vi "Periodic Tasks.vi"(8 "error in":errorcluster) -> ()   [LabVIEW 2015]
doc: "This VI runs in parallel to other tasks. It can contain as many user-defined periodic loops as you need. These can carry out PID or other sorts of timed response."
uses:
  Device Refnums.ctl
  Drive Base - Controlled Mode - TypeDef.ctl
  Drive Base Mode.ctl
  Shooter Control.ctl
  Arm Mode TypeDef.ctl
  <vilib>/Rock Robotics/WPI/Solenoid/WPI_SolenoidValue.ctl
  Operator-Interface-Control-Board.git/trunk/LabVIEW/LED_Output_TypeDef.ctl
  Operator-Interface-Control-Board.git/trunk/LabVIEW/PWM_Output_TypeDef.ctl
  <vilib>/Rock Robotics/WPI/CAN/TalonSRX/WPI_CANTalonSRX_APIControlMode.ctl
  <vilib>/Rock Robotics/WPI/Utilities/WPI_GetSetVariantRefNum.vi
  Global Variables.vi
  <vilib>/Rock Robotics/Network Tables/NT Write Number.vi
  <vilib>/Rock Robotics/Network Tables/NT Read Number.vi
  <vilib>/addons/control/pid/pid.llb/PID (DBL).vi
  <vilib>/Rock Robotics/Network Tables/NT Write Numeric Array.vi
  <vilib>/Rock Robotics/WPI/Solenoid/WPI_SolenoidSetEnum.vi
  <vilib>/Rock Robotics/Network Tables/NT Write String.vi
  <vilib>/Rock Robotics/Network Tables/NT Write Boolean.vi
  <vilib>/Rock Robotics/WPI/Ultrasonic/WPI_SonarMB1010DigitalRefNum Registry Get.vi
  <vilib>/Rock Robotics/WPI/Ultrasonic/WPI_SonarMB1010DigitalGetRange.vi
  <vilib>/Utility/config.llb/Read Key (String).vi
  <vilib>/Utility/config.llb/Read Key (Boolean).vi
  <vilib>/Utility/config.llb/Read Key (Double).vi
  <vilib>/Rock Robotics/Network Tables/NT Write Raw.vi
  <vilib>/Rock Robotics/Network Tables/NT Write Boolean Array.vi
  <vilib>/Rock Robotics/Network Tables/NT Write String Array.vi
  ADIS16448-RoboRIO-Driver.git/trunk/LabVIEW/ADI MXP IMU/FRC ADI MXP IMU.lvlib
  <vilib>/addons/control/pid/NI_PID_pid.lvlib
  <vilib>/Utility/config.llb/NI_LVConfig.lvlib
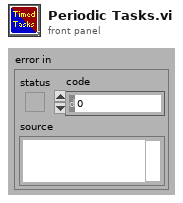
[diagram p1: front panel]
types:
  T1 = typedef "Device Refnums.ctl" = string
  T2 = typedef "Shooter Control.ctl" = cluster{"Fire":bool, "Open Claw":bool}
  T3 = typedef "Drive Base Mode.ctl" = enum16{"Disabled", "Controlled - Arcade", "Controlled - Tank", "Braked", "GRIP", "Encoder", "IMU", "Distance"}
  T4 = typedef "Drive Base - Controlled Mode - TypeDef.ctl" = cluster{"Drive Base Mode":T3, "Arcade":cluster{"y":dbl, "x":dbl}, "Tank":cluster{"Left":dbl, "Right":dbl}, "Target Encoder Value":cluster{"Left":dbl, "Right":dbl}, "Target IMU Angle":dbl, "Distance":dbl, "Target GRIP Area":dbl}
  T5 = typedef "WPI_EncoderDevRef.ctl" = cluster{"DevStatus":errorcluster, "EncoderIndex":T6, "CounterIndex":T7, "DistancePerCount":dbl, "Decoding Type":T8}
  T6 = typedef "FPGA_EncoderIdx.ctl" = enum8{"Enc 0", "Enc 1", "Enc 2", "Enc 3", "Enc 4", "Enc 5", "Enc 6", "Enc 7", "Invalid"}
  T7 = typedef "FPGA_CounterCtrSystemIndex.ctl" = enum8{"Ctr 0", "Ctr 1", "Ctr 2", "Ctr 3", "Ctr 4", "Ctr 5", "Ctr 6", "Ctr 7", "Invalid"}
  T8 = typedef "WPI_EncoderType.ctl" = enum16{"1x", "2x", "4x"}
  T9 = typedef "WPI_RobotDriveDevRef.ctl" = cluster{"DevStatus":errorcluster, "Motors[]":T10[], "Square Inputs":bool, "Max Output":dbl}
  T10 = typedef "WPI_MotorControlDeviceRef.ctl" = cluster{"DeviceStatus":errorcluster, "Type":T11, "PWM":cluster{"PWM Channel":T12, "DeadBand":T13}, "CAN":cluster{"Device Number":u8, "Control Mode":T14, "Semaphore":T15, "Max Vout":dbl, "TalonSRX Control Mode":T16}, "Invert":bool}
  T11 = typedef "WPI_MotorControlType.ctl" = enum16{"PWM", "CAN", "CANTalonSRX"}
  T12 = typedef "FPGA_DIOPWMChannel.ctl" = enum8{"PWM 0", "PWM 1", "PWM 2", "PWM 3", "PWM 4", "PWM 5", "PWM 6", "PWM 7", "PWM 8", "PWM 9", "PWM MXP 0", "PWM MXP 1", "PWM MXP 2", "PWM MXP 3", "PWM MXP 4", "PWM MXP 5", "PWM MXP 6", "PWM MXP 7", "PWM MXP 8", "PWM MXP 9", "Invalid"}
  T13 = typedef "WPI_PWMDeadband.ctl" = cluster{"Name":string, "maxPositivePwm":i32, "minPositivePwm":i32, "centerPwm":i32, "maxNegativePwm":i32, "minNegativePwm":i32, "angularRange":u16}
  T14 = typedef "WPI_CANJaguar_ControlMode.ctl" = enum8{"Percent VBus", "Current", "Speed", "Position", "Voltage"}
  T15 = typedef "Semaphore RefNum" = refnum<k1>
  T16 = typedef "WPI_CANTalonSRX_APIControlMode.ctl" = enum8{"Percent VBus", "Speed", "Position", "Slave", "Unchanged / Invalid", "Voltage Compensation", "Current", "Motion Profile"}
  T17 = typedef "WPI_SonarMB1010DigitalDeviceRef.ctl" = cluster{"CounterDevRef":T18, "Scaling factor (s/in)":dbl}
  T18 = typedef "WPI_CounterDevRef.ctl" = cluster{"DevStatus":errorcluster, "CntIndex":T7}
  T19 = typedef "FRC ADI MXP IMU.lvlib/WPI_AnalogDevicesIMUInterruptDevRef.ctl" = cluster{"SimpleGyroDevRef":T20, "InterruptRef":T22}
  T20 = typedef "FRC ADI MXP IMU.lvlib/WPI_AnalogDevicesIMUDevRef.ctl" = cluster{"DevStatus":errorcluster, "Handle":i32, "SPI Bus":T21, "Device Found":bool, "Sample Rate":dbl, "Device Ready":bool, "Yaw Axis":enum16{"X", "Y", "Z"}, "AHRS Algorithm":enum16{"Complementary", "Madgwick"}}
  T21 = typedef "spi_bus.ctl" = enum16{"SPI On-Board, CS0", "SPI On-Board, CS1", "SPI On-Board, CS2", "SPI On-Board, CS3", "SPI MXP", "Invalid"}
  T22 = typedef "WPI_InterruptRef.ctl" = cluster{"DevStatus":errorcluster, "InterruptIndex":T23}
  T23 = typedef "FPGA_InterruptIndex.ctl" = enum8{"0", "1", "2", "3", "4", "5", "6", "7", "Invalid"}
  T24 = typedef "WPI_AnalogChannelDevRef.ctl" = cluster{"DevStatus":errorcluster, "Analog Channel":T25}
  T25 = typedef "FPGA_AIChannel.ctl" = enum8{"AI 0", "AI 1", "AI 2", "AI 3", "AI MXP 0", "AI MXP 1", "AI MXP 2", "AI MXP 3", "Invalid"}
  T26 = typedef "Switch_Input_TypeDef.ctl" = cluster{"SW 0":bool, "SW 1":bool, "SW 2":bool, "SW 3":bool, "SW 4":bool, "SW 5":bool, "SW 6":bool, "SW 7":bool, "SW 8":bool, "SW 9":bool, "SW 10":bool, "SW 11":bool, "SW 12":bool, "SW 13":bool, "SW 14":bool, "SW 15":bool}
  T27 = typedef "GRIP Contours Report.ctl" = cluster{"area":dbl, "centerX":dbl, "centerY":dbl, "width":dbl, "height":dbl, "solidity":dbl}
  T28 = cluster{"proportional gain (Kc)":dbl, "integral time (Ti, min)":dbl, "derivative time (Td, min)":dbl}
  T29 = typedef "IMU AHRS TypeDef.ctl" = cluster{"Pitch":dbl, "Roll":dbl, "Yaw":dbl}
  T30 = typedef "WPI_SolenoidDevRef.ctl" = cluster{"DevStatus":errorcluster, "Pneumatics Control Module":u8, "Forward Solenoid Channel":T31, "Reverse Solenoid Channel":T31}
  T31 = typedef "WPI_SolenoidChannel.ctl" = enum8{"Solenoid 0", "Solenoid 1", "Solenoid 2", "Solenoid 3", "Solenoid 4", "Solenoid 5", "Solenoid 6", "Solenoid 7", "Invalid"}
  T32 = typedef "WPI_SolenoidValue.ctl" = enum16{"Off", "On", "Forward", "Reverse"}
  T33 = typedef "WPI_SwitchDevRef.ctl" = cluster{"DevStatus":errorcluster, "DIO Channel":T34, "CntIndex":T7, "Normally Closed":bool}
  T34 = typedef "FPGA_DIOChannel.ctl" = enum8{"DIO 0", "DIO 1", "DIO 2", "DIO 3", "DIO 4", "DIO 5", "DIO 6", "DIO 7", "DIO 8", "DIO 9", "DIO MXP 0", "DIO MXP 1", "DIO MXP 2", "DIO MXP 3", "DIO MXP 4", "DIO MXP 5", "DIO MXP 6", "DIO MXP 7", "DIO MXP 8", "DIO MXP 9", "DIO MXP 10", "DIO MXP 11", "DIO MXP 12", "DIO MXP 13", "DIO MXP 14", "DIO MXP 15", "Invalid"}
  T35 = typedef "NI_LVConfig.lvlib/Config Data RefNum.ctl" = refnum<k1>
  T36 = typedef "Arm Mode TypeDef.ctl" = enum16{"Unknown", "Disabled", "Locked", "Shoot Batter", "Shoot Close", "Cross Defense", "Human Player Load", "Low Bar / Goal", "Manual"}
  T37 = typedef "Arm Notifier TypeDef.ctl" = cluster{"Arm Mode":T36, "Manual Arm Angle":dbl}
  T38 = typedef "PWM_Output_TypeDef.ctl" = cluster{"PWM 0":u8, "PWM 1":u8, "PWM 2":u8, "PWM 3":u8, "PWM 4":u8, "PWM 5":u8, "PWM 6":u8, "PWM 7":u8, "PWM 8":u8, "PWM 9":u8, "PWM 10":u8}
  T39 = typedef "LED_Output_TypeDef.ctl" = cluster{"LED 0":bool, "LED 1":bool, "LED 2":bool, "LED 3":bool, "LED 4":bool, "LED 5":bool, "LED 6":bool, "LED 7":bool, "LED 8":bool, "LED 9":bool, "LED 10":bool, "LED 11":bool, "LED 12":bool, "LED 13":bool, "LED 14":bool, "LED 15":bool}
  T40 = typedef "Arm Mode LEDs.ctl" = cluster{"Shoot Batter":bool, "Shoot Close":bool, "Shoot Far":bool, "Low Bar / Goal":bool, "Human Player Load":bool, "Manual":bool}
  T41 = typedef "Analog_Input_TypeDef.ctl" = cluster{"ANA 0":u8, "ANA 1":u8, "ANA 2":u8, "ANA 3":u8, "ANA 4":u8, "ANA 5":u8, "ANA 6":u8, "ANA 7":u8, "ANA 8":u8, "ANA 9":u8, "ANA 10":u8, "ANA 11":u8, "ANA 12":u8, "ANA 13":u8, "ANA 14":u8, "ANA 15":u8}
  T42 = typedef "Autonomous Mode.ctl" = enum16{"Off", "Cross Defense", "Shoot A/B", "Shoot C/D", "Shoot E"}
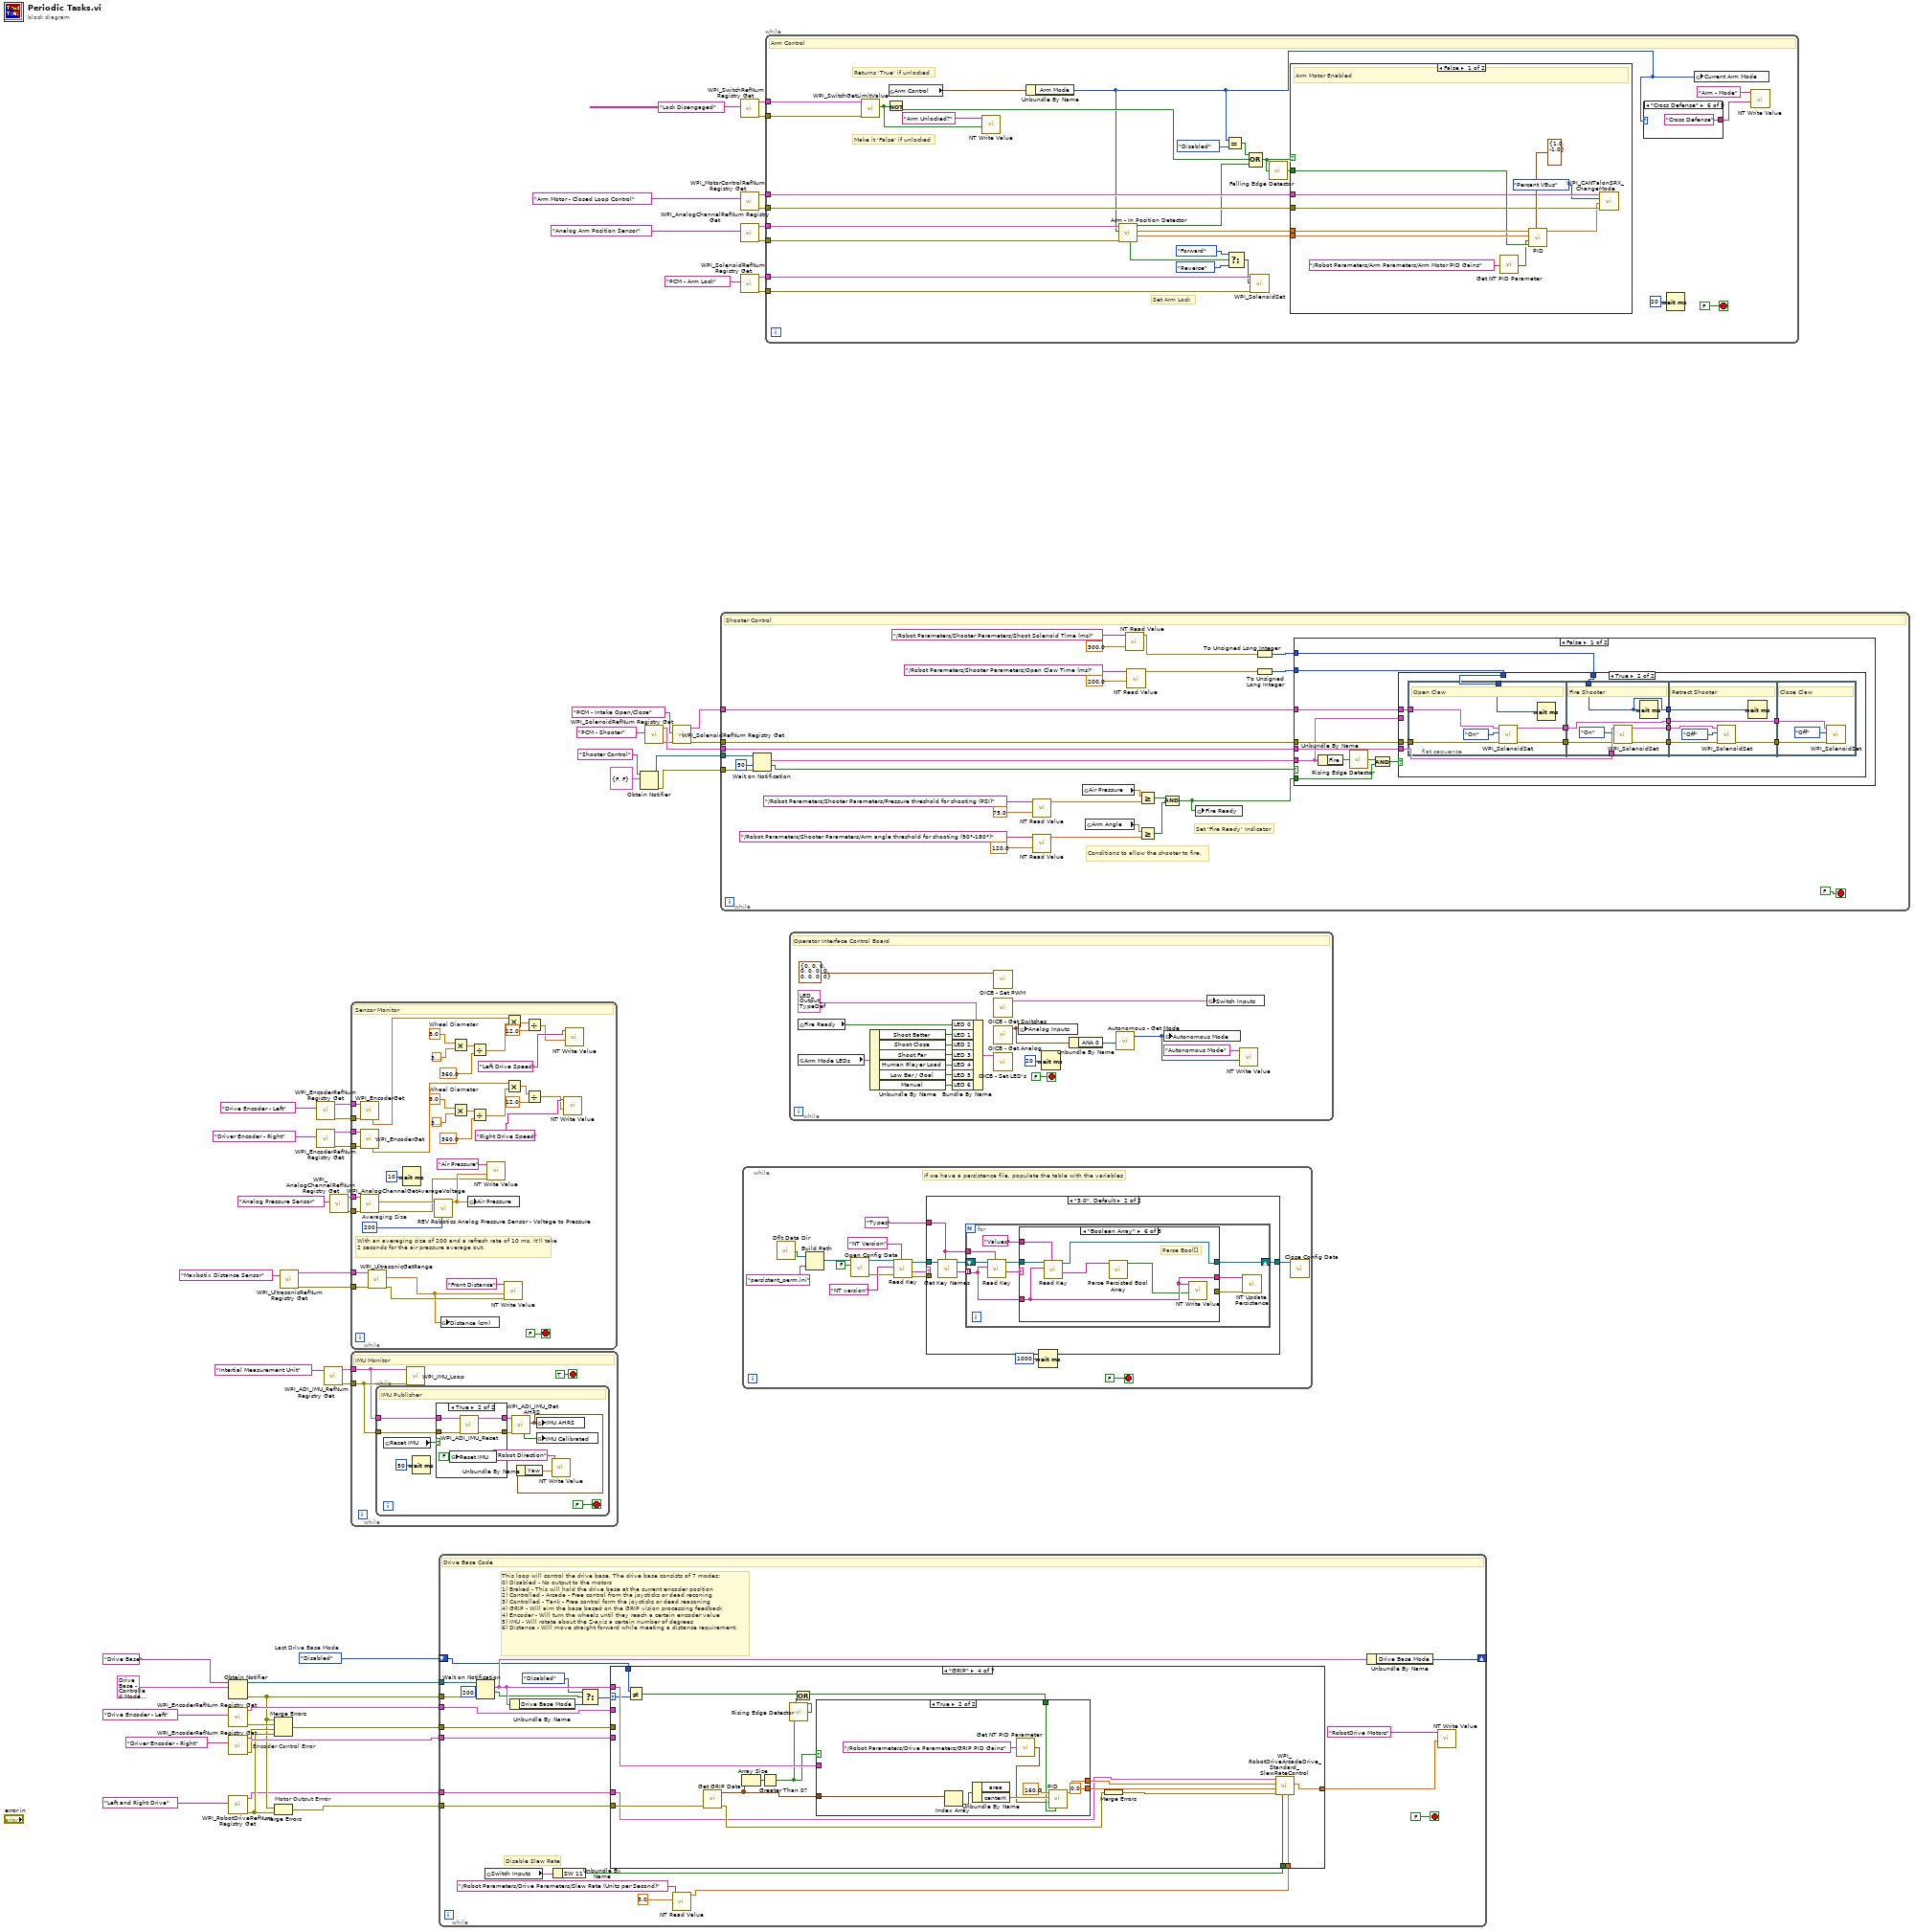
[diagram p0: block diagram]
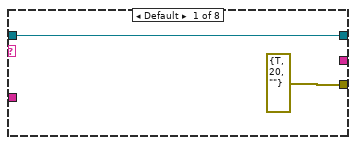
[diagram p3: hidden frame]
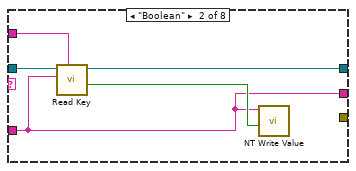
[diagram p4: hidden frame]
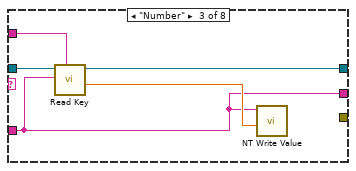
[diagram p5: hidden frame]
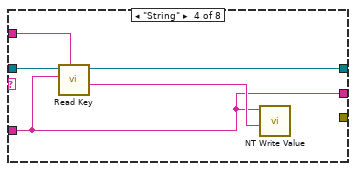
[diagram p6: hidden frame]
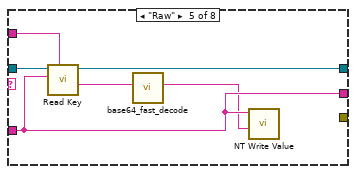
[diagram p7: hidden frame]
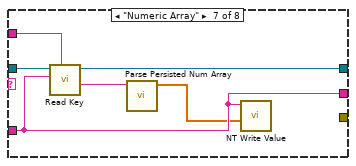
[diagram p8: hidden frame]
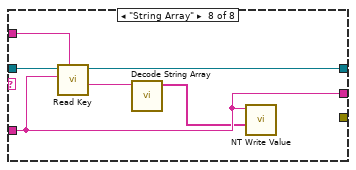
[diagram p9: hidden frame]
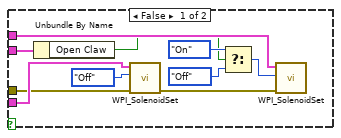
[diagram p11: hidden frame]
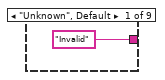
[diagram p13: hidden frame]
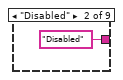
[diagram p14: hidden frame]
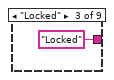
[diagram p15: hidden frame]
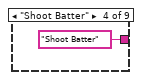
[diagram p16: hidden frame]
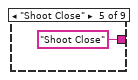
[diagram p17: hidden frame]
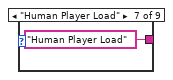
[diagram p18: hidden frame]
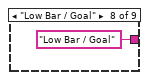
[diagram p19: hidden frame]
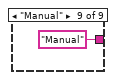
[diagram p20: hidden frame]
diagram:
  w37 = Drive_Base_Mode."Disabled"  # Last Drive Base Mode
  n1 = Obtain Notifier(name (unnamed)="Drive Base", notification data type=T4 {"Drive Base Mode"=enum."Disabled", "Arcade"={"y"=0.0, "x"=0.0}, "Tank"={"Left"=0.0, "Right"=0.0}, "Target Encoder Value"={"Left"=0.0, "Right"=0.0}, "Target IMU Angle"=0.0, "Distance"=0.0, "Target GRIP Area"=0.0}) -> (notifier out=w50:refnum<notifier>, error out=w40:errorcluster)  [unwired: 2 in, 1 out]
  n2 = call <vilib>:"WPI_EncoderRefNum Registry Get.vi"("refnum name"=T1 "Drive Encoder - Left" ("Device Name")) -> ("error out"=w44:errorcluster, "EncoderDevRef"=w47:T5)  [unwired: 9 in]
  n3 = call <vilib>:"WPI_EncoderRefNum Registry Get.vi"("refnum name"=T1 "Driver Encoder - Right" ("Device Name")) -> ("error out"=w43:errorcluster, "EncoderDevRef"=w46:T5)  [unwired: 9 in]
  n4 = call <vilib>:"WPI_RobotDriveRefNum Registry Get.vi"("refnum name"=T1 "Left and Right Drive" ("Device Name")) -> ("error out"=w41:errorcluster, "RobotDriveDevRef"=w39:T9)  [unwired: 1 in, 8 out]
  n5 = Merge Errors "Encoder Control Error"(w40, w44, w43, w41) -> (w42:errorcluster)
  n6 = Merge Errors "Motor Output Errror"(w40, w41) -> (w38:errorcluster)
  n7 = call-poly <vilib>:"WPI_UltrasonicRefNum Registry Get.vi"("refnum name"=T1 "Maxbotix Distance Sensor" ("Device Name")) -> ("error out"=w7:errorcluster, "SonarMB1010DigitalDevRef"=w8:T17)  [unwired: 9 in]
  n8 = call <vilib>:"WPI_EncoderRefNum Registry Get.vi"("refnum name"=T1 "Drive Encoder - Left" ("Device Name")) -> ("error out"=w3:errorcluster, "EncoderDevRef"=w4:T5)  [unwired: 9 in]
  n9 = call <vilib>:"WPI_EncoderRefNum Registry Get.vi"("refnum name"=T1 "Driver Encoder - Right" ("Device Name")) -> ("error out"=w1:errorcluster, "EncoderDevRef"=w2:T5)  [unwired: 9 in]
  n10 = call "WPI_ADI_IMU_RefNum Registry Get.vi"("refnum name"=T1 "Intertial Measurement Unit" ("Device Name")) -> ("error out"=w13:errorcluster, "ADI IMU Interrupt DevRef"=w12:T19)  [unwired: 9 in]
  n11 = call <vilib>:"WPI_AnalogChannelRefNum Registry Get.vi"("refnum name"=T1 "Analog Pressure Sensor" ("Device Name")) -> ("error out"=w18:errorcluster, "AIDeviceRef"=w19:T24)  [unwired: 9 in]
  n12 = while {
    tunnel: w19 -> [w87]
    tunnel: w18 -> [w86]
    tunnel: w8 -> [w82]
    tunnel: w7 -> [w83]
    tunnel: w4 -> [w77]
    tunnel: w3 -> [w76]
    tunnel: w2 -> [w75]
    tunnel: w1 -> [w74]
    stop <- FALSE stop-if-true
    w67 = 8.0  # Wheel Diameter
    w70 = 8.0  # Wheel Diameter
    w85 = 200  # Averaging Size
    # "With an averaging size of 200 and a refresh rate of 10 ms, it'll take 2 seconds for the air pressure average out."
    # "Sensor Monitor"
    n13 = call <vilib>:"WPI_AnalogChannelGetAverageVoltage.vi"("error in (no error)"=w86, "AIDeviceRef"=w87) -> ("error out"=w79:errorcluster, "Voltage"=w89:dbl)  [unwired: 7 in, 1 out]
    n14 = call <vilib>:"WPI_EncoderGet.vi"("error in (no error)"=w76, "EncoderDevRef"=w77) -> ("Rate"=w63:dbl)  [unwired: 4 in, 5 out]
    n15 = call <vilib>:"WPI_EncoderGet.vi"("error in (no error)"=w74, "EncoderDevRef"=w75) -> ("Rate"=w62:dbl)  [unwired: 4 in, 5 out]
    n16 = call-poly <vilib>:"WPI_UltrasonicGetRange.vi"("error in"=w83, "SonarMB1010DigitalDevRef"=w82) -> ("error out"=w80:errorcluster, "Distance"=w78:dbl)  [unwired: 7 in, 1 out]
    n17 = Wait (ms)(milliseconds to wait=u32 10) -> ()  [unwired: 1 out]
    n18 = call "REV Robotics Analog Pressure Sensor - Voltage to Pressure.vi"("Averaging Size"=w85, "Voltage (V)"=w89) -> ("Pressure (PSI)"=w84:dbl)  [unwired: 7 in]
    n19 = global write "Global Variables.vi" "Distance (cm)"(w78) -> ()
    n20 = Multiply(x=w67, y=3.141592653589793) -> (x*y=w66:dbl)
    n21 = Multiply(x=w70, y=3.141592653589793) -> (x*y=w71:dbl)
    n22 = global write "Global Variables.vi" "Air Pressure"(w84) -> ()
    n23 = Divide(x=w66, y=360.0) -> (x/y=w64:dbl)
    n24 = Divide(x=w71, y=360.0) -> (x/y=w73:dbl)
    n25 = call-poly <vilib>:"NT Write Value.vi"("error in"=w79, "Numeric"=w84, "Name"="Air Pressure") -> ()  [unwired: 8 in, 1 out]
    n26 = call-poly <vilib>:"NT Write Value.vi"("error in"=w80, "Numeric"=w78, "Name"="Front Distance") -> ()  [unwired: 8 in, 1 out]
    n27 = Multiply(x=w63, y=w64) -> (x*y=w61:dbl)
    n28 = Multiply(x=w62, y=w73) -> (x*y=w58:dbl)
    n29 = Divide(x=w61, y=12.0) -> (x/y=w54:dbl)
    n30 = Divide(x=w58, y=12.0) -> (x/y=w55:dbl)
    n31 = call-poly <vilib>:"NT Write Value.vi"("Numeric"=w55, "Name"="Right Drive Speed") -> ()  [unwired: 9 in, 1 out]
    n32 = call-poly <vilib>:"NT Write Value.vi"("Numeric"=w54, "Name"="Left Drive Speed") -> ()  [unwired: 9 in, 1 out]
  }
  n33 = while {
    tunnel: w13 -> [w94]
    tunnel: w12 -> [w93]
    stop <- TRUE stop-if-true
    # "IMU Monitor"
    n34 = while {
      tunnel: w94 -> [w101]
      tunnel: w93 -> [w102]
      stop <- FALSE stop-if-true
      # "IMU Publisher"
      n35 = global read "Global Variables.vi" "Reset IMU"() -> (w103:bool)
      n36 = Wait (ms)(milliseconds to wait=u32 50) -> ()  [unwired: 1 out]
      n37 = case shown="True" w103 {
        tunnel: w102 -> [w107 w111]
        tunnel: w101 -> [w106 w110]
        tunnel: [w107 w109] -> w99
        tunnel: [w106 w108] -> w98
        frame False {
        }
        frame True {
          n38 = global write "Global Variables.vi" "Reset IMU"(FALSE ("Reset IMU")) -> ()
          n39 = call "WPI_ADI_IMU_Reset.vi"("error in"=w110, "ADI IMU Interrupt DevRef"=w111) -> ("error out"=w108:errorcluster, "ADI IMU Interrupt DevRef Out"=w109:T19)  [unwired: 8 in]
        }
      }
      n40 = call "WPI_ADI_IMU_Get AHRS.vi"("error in"=w98, "ADI IMU Interrupt DevRef"=w99) -> ("IMU AHRS"=w96:cluster{"Pitch":dbl, "Roll":dbl, "Yaw":dbl}, "Sensor Ready Out"=w100:bool)  [unwired: 5 in, 3 out]
      n41 = Unbundle By Name(w96) -> ("Yaw"=w95:dbl)
      n42 = global write "Global Variables.vi" "IMU AHRS"(w96) -> ()
      n43 = global write "Global Variables.vi" "IMU Calibrated"(w100) -> ()
      n44 = call-poly <vilib>:"NT Write Value.vi"("Numeric"=w95, "Name"="Robot Direction") -> ()  [unwired: 9 in, 1 out]
    }
    n45 = call "WPI_IMU_Loop.vi"("error in"=w94, "ADI IMU Interrupt DevRef"=w93) -> ()  [unwired: 8 in, 2 out]
  }
  n46 = while {
    tunnel: w39 -> [w134]
    tunnel: w50 -> [w133]
    tunnel: w40 -> [w132]
    tunnel: w47 -> [w131]
    tunnel: w46 -> [w130]
    tunnel: w42 -> [w128]
    tunnel: w38 -> [w129]
    shift-right: [w127] -> _
    shift-left: w37 -> [w125]
    stop <- FALSE stop-if-true
    # "Disable Slew Rate"
    # "This loop will control the drive base. The drive base consists of 7 modes:\n0) Disabled - No output to the motors\n1) Braked - This will hold the drive base at the current encoder position\n2) Controlled - Arcade - Free control from the joysticks or dead reconing\n3) Controlled - Tank - Free control form the joysticks or dead reaconing\n4) GRIP - Will aim the base based on the GRIP vision processing feedback\n4) Encoder - Will turn the wheels until they reach a certain encoder value\n5) IMU - Will rotate about the Z-axis a certain number of degrees\n6) Distance - Will move straight forward while meeting a distance requirement."
    # "Drive Base Code"
    n47 = Wait on Notification(notifier=w133, timeout in ms (-1)=200, error in (no error)=w132) -> (notification=w126:T4, timed out?=w123:bool)  [unwired: 1 in, 2 out]
    n48 = global read "Global Variables.vi" "Switch Inputs"() -> (w117:T26)
    n49 = Unbundle By Name(w126) -> ("Drive Base Mode"=w122:T3)
    n50 = Unbundle By Name(w117) -> ("SW 11"=w116:bool)
    n51 = Select(t=Drive_Base_Mode."Disabled", s=w123, f=w122) -> (s? t:f=w120:T3)
    n52 = call-poly <vilib>:"NT Read Value.vi"("Default Value"=3.0, "Name"="/Robot Parameters/Drive Parameters/Slew Rate (Units per Second)") -> ("Numeric"=w115:dbl)  [unwired: 8 in, 1 out]
    n53 = case shown="\"GRIP\"" w120 {
      selector: w120 -> [_ _ _ w172 w211 w241 w260]
      tunnel: w134 -> [w141 w149 w154 w160 w194 w238 w259]
      tunnel: w126 -> [_ w147 w153 w175 w198 w237 _]
      tunnel: w131 -> [_ _ _ _ w210 _ w265]
      tunnel: w130 -> [_ _ _ _ w209 _ w264]
      tunnel: w129 -> [w139 w148 w155 w174 _ w236 _]
      tunnel: w128 -> [_ _ _ _ w191 _ w257]
      tunnel: w125 -> [_ _ _ w171 w212 w240 w261]
      tunnel: [w138 w144 w152 w164 w193 w231 w258] -> w118
      tunnel: w116 -> [w137 w143 w151 w159 w190 w227 w256]
      tunnel: w115 -> [w136 w142 w150 w158 w189 w226 w255]
      frame "Disabled", Default {
        w140 = 0.0
        n54 = call "WPI_RobotDriveTankDrive_SlewRateControl.vi"("Slew Rate (Unit/Sec)"=w136, "Disable Slew"=w137, "error in (no error)"=w139, "Right axis value"=w140, "Left axis value"=w140, "RobotDriveDevRef"=w141) -> ("Motor Values"=w138:dbl[])  [unwired: 3 in, 2 out]
      }
      frame "Controlled - Arcade" {
        n55 = Unbundle By Name(w147) -> ("Arcade.x"=w145:dbl, "Arcade.y"=w146:dbl)
        n56 = call "WPI_RobotDriveArcadeDrive_Standard_SlewRateControl.vi"("Slew Rate (Unit/Sec)"=w142, "Disable Slew"=w143, "error in (no error)"=w148, "Y axis value"=w146, "X axis value"=w145, "RobotDriveDevRef"=w149) -> ("Motor Values"=w144:dbl[])  [unwired: 3 in, 2 out]
      }
      frame "Controlled - Tank" {
        n57 = Unbundle By Name(w153) -> ("Tank.Left"=w157:dbl, "Tank.Right"=w156:dbl)
        n58 = call "WPI_RobotDriveTankDrive_SlewRateControl.vi"("Slew Rate (Unit/Sec)"=w150, "Disable Slew"=w151, "error in (no error)"=w155, "Right axis value"=w156, "Left axis value"=w157, "RobotDriveDevRef"=w154) -> ("Motor Values"=w152:dbl[])  [unwired: 3 in, 2 out]
      }
      frame "GRIP" {
        n59 = Not Equal?(x=w171, y=w172) -> (x != y?=w170:bool)
        n60 = call "Get GRIP Data.vi"("error in (no error)"=w174) -> ("error out"=w173:errorcluster, "ContoursReport"=w169:T27[])  [unwired: 8 in, 1 out]
        n61 = Array Size(array=w169) -> (size(s)=w168:i32)
        n62 = Greater Than 0?(x=w168) -> (x > 0?=w167:bool)
        n63 = call "Rising Edge Detector.vi"("Input"=w167) -> ("Rising Edge Detected"=w165:bool)
        n64 = Or(x=w170, y=w165) -> (x .or. y?=w166:bool)
        n65 = case shown="True" w167 {
          tunnel: w175 -> [_ _]
          tunnel: w166 -> [_ w183]
          tunnel: [0.0 ("output") 0.0 ("output")] -> w162
          tunnel: [0.0 ("output") w182] -> w163
          tunnel: w169 -> [_ w181]
          frame False {
          }
          frame True {
            n66 = Index Array(array=w181) -> (element=w186:T27)  [unwired: 1 in]
            n67 = Unbundle By Name(w186) -> ("centerX"=w185:dbl)  [unwired: 1 out]
            n68 = call "Get NT PID Parameter.vi"("NT Path"="/Robot Parameters/Drive Parameters/GRIP PID Gains") -> ("PID Gains"=w178:T28)
            n69 = call-poly <vilib>:"PID.vi"("reinitialize? (F)"=w183, "PID gains"=w178, "process variable"=w185, "setpoint"=160.0) -> ("output"=w182:dbl)  [unwired: 6 in, 1 out]
          }
        }
        n70 = Merge Errors(w173) -> (w161:errorcluster)
        n71 = call "WPI_RobotDriveArcadeDrive_Standard_SlewRateControl.vi"("Slew Rate (Unit/Sec)"=w158, "Disable Slew"=w159, "error in (no error)"=w161, "Y axis value"=w162, "X axis value"=w163, "RobotDriveDevRef"=w160) -> ("Motor Values"=w164:dbl[])  [unwired: 3 in, 2 out]
      }
      frame "Encoder" {
        w208 = cluster{"output high":dbl, "output low":dbl} {"output high"=1.0, "output low"=-1.0}  # output range
        n72 = Not Equal?(x=w212, y=w211) -> (x != y?=w192:bool)
        n73 = case shown="True" w192 {
          tunnel: w210 -> [w215 w223]
          tunnel: w209 -> [w214 w222]
          tunnel: [w215 w221] -> w206
          tunnel: [w214 w220] -> w205
          tunnel: [w213 w219] -> w207
          tunnel: w191 -> [w213 w216]
          frame False {
          }
          frame True {
            # "Reset Encoders"
            n74 = call <vilib>:"WPI_EncoderReset.vi"("error in (no error)"=w216, "EncoderDevRef"=w223) -> ("error out"=w218:errorcluster, "EncoderDevRef"=w221:T5)  [unwired: 8 in]
            n75 = call <vilib>:"WPI_EncoderReset.vi"("error in (no error)"=w216, "EncoderDevRef"=w222) -> ("error out"=w217:errorcluster, "EncoderDevRef"=w220:T5)  [unwired: 8 in]
            n76 = Merge Errors(w218, w217) -> (w219:errorcluster)
          }
        }
        n77 = call <vilib>:"WPI_EncoderGet.vi"("error in (no error)"=w207, "EncoderDevRef"=w205) -> ("error out"=w196:errorcluster, "Distance"=w203:dbl)  [unwired: 4 in, 4 out]
        n78 = call <vilib>:"WPI_EncoderGet.vi"("error in (no error)"=w207, "EncoderDevRef"=w206) -> ("error out"=w197:errorcluster, "Distance"=w204:dbl)  [unwired: 4 in, 4 out]
        n79 = Unbundle By Name(w198) -> ("Target Encoder Value.Right"=w199:dbl)
        n80 = Unbundle By Name(w198) -> ("Target Encoder Value.Left"=w200:dbl)
        n81 = Merge Errors(w197, w196) -> (w195:errorcluster)
        n82 = call "Get NT PID Parameter.vi"("NT Path"="/Robot Parameters/Drive Parameters/Encoder PID Gains") -> ("PID Gains"=w187:T28)
        n83 = call-poly <vilib>:"PID.vi"("reinitialize? (F)"=w192, "output range"=w208, "PID gains"=w187, "process variable"=w204, "setpoint"=w200) -> ("output"=w202:dbl)  [unwired: 5 in, 1 out]
        n84 = call-poly <vilib>:"PID.vi"("reinitialize? (F)"=w192, "output range"=w208, "PID gains"=w187, "process variable"=w203, "setpoint"=w199) -> ("output"=w201:dbl)  [unwired: 5 in, 1 out]
        n85 = call "WPI_RobotDriveTankDrive_SlewRateControl.vi"("Slew Rate (Unit/Sec)"=w189, "Disable Slew"=w190, "error in (no error)"=w195, "Right axis value"=w201, "Left axis value"=w202, "RobotDriveDevRef"=w194) -> ("Motor Values"=w193:dbl[])  [unwired: 3 in, 2 out]
      }
      frame "IMU" {
        n86 = Not Equal?(x=w240, y=w241) -> (x != y?=w230:bool)
        n87 = global read "Global Variables.vi" "IMU AHRS"() -> (w229:T29)
        n88 = global read "Global Variables.vi" "IMU Calibrated"() -> (w228:bool)
        n89 = global write "Global Variables.vi" "Reset IMU"(w230) -> ()
        n90 = call "Get NT PID Parameter.vi"("NT Path"="/Robot Parameters/Drive Parameters/IMU PID Gains") -> ("PID Gains"=w224:T28)
        n91 = Not(x=w230) -> (.not. x?=w234:bool)
        n92 = And(x=w228, y=w234) -> (x .and. y?=w233:bool)
        n93 = feedback-in #1(w233) -> ()
        n94 = feedback #1() -> (w232:bool)  [unwired: 1 in]
        n95 = case shown="True" w233 {
          selector: w233 -> [_ w247]
          tunnel: w229 -> [_ w252]
          tunnel: w237 -> [_ w250]
          tunnel: [0.0 ("Y axis value") w244] -> w235
          tunnel: w232 -> [_ w248]
          tunnel: w224 -> [_ w243]
          frame False {
          }
          frame True {
            w245 = cluster{"output high":dbl, "output low":dbl} {"output high"=1.0, "output low"=-1.0}  # output range
            n96 = Unbundle By Name(w250) -> ("Target IMU Angle"=w249:dbl)
            n97 = Unbundle By Name(w252) -> ("Yaw"=w251:dbl)
            n98 = Greater?(x=w247, y=w248) -> (0:w246:bool)
            n99 = call-poly <vilib>:"PID.vi"("reinitialize? (F)"=w246, "output range"=w245, "PID gains"=w243, "process variable"=w251, "setpoint"=w249) -> ("output"=w244:dbl)  [unwired: 5 in, 1 out]
          }
        }
        n100 = call "WPI_RobotDriveArcadeDrive_Standard_SlewRateControl.vi"("Slew Rate (Unit/Sec)"=w226, "Disable Slew"=w227, "error in (no error)"=w236, "Y axis value"=0.0, "X axis value"=w235, "RobotDriveDevRef"=w238) -> ("Motor Values"=w231:dbl[])  [unwired: 3 in, 2 out]
      }
      frame "Braked" {
        w277 = cluster{"output high":dbl, "output low":dbl} {"output high"=1.0, "output low"=-1.0}  # output range
        n101 = Not Equal?(x=w261, y=w260) -> (x != y?=w275:bool)
        n102 = case shown="True" w275 {
          tunnel: [w280 w288] -> w274
          tunnel: [w279 w287] -> w273
          tunnel: [w278 w286] -> w276
          tunnel: w265 -> [w280 w283]
          tunnel: w264 -> [w279 w282]
          tunnel: w257 -> [w278 w281]
          frame False {
          }
          frame True {
            # "Reset Encoders"
            n103 = call <vilib>:"WPI_EncoderReset.vi"("error in (no error)"=w281, "EncoderDevRef"=w283) -> ("error out"=w285:errorcluster, "EncoderDevRef"=w288:T5)  [unwired: 8 in]
            n104 = call <vilib>:"WPI_EncoderReset.vi"("error in (no error)"=w281, "EncoderDevRef"=w282) -> ("error out"=w284:errorcluster, "EncoderDevRef"=w287:T5)  [unwired: 8 in]
            n105 = Merge Errors(w285, w284) -> (w286:errorcluster)
          }
        }
        n106 = call "Get NT PID Parameter.vi"("NT Path"="/Robot Parameters/Drive Parameters/Encoder PID Gains") -> ("PID Gains"=w254:T28)
        n107 = call <vilib>:"WPI_EncoderGet.vi"("error in (no error)"=w276, "EncoderDevRef"=w273) -> ("error out"=w267:errorcluster, "Distance"=w271:dbl)  [unwired: 4 in, 4 out]
        n108 = call <vilib>:"WPI_EncoderGet.vi"("error in (no error)"=w276, "EncoderDevRef"=w274) -> ("error out"=w268:errorcluster, "Distance"=w272:dbl)  [unwired: 4 in, 4 out]
        n109 = Merge Errors(w268, w267) -> (w266:errorcluster)
        n110 = call-poly <vilib>:"PID.vi"("reinitialize? (F)"=w275, "output range"=w277, "PID gains"=w254, "process variable"=w272, "setpoint"=0.0) -> ("output"=w270:dbl)  [unwired: 5 in, 1 out]
        n111 = call-poly <vilib>:"PID.vi"("reinitialize? (F)"=w275, "output range"=w277, "PID gains"=w254, "process variable"=w271, "setpoint"=0.0) -> ("output"=w269:dbl)  [unwired: 5 in, 1 out]
        n112 = call "WPI_RobotDriveTankDrive_SlewRateControl.vi"("Slew Rate (Unit/Sec)"=w255, "Disable Slew"=w256, "error in (no error)"=w266, "Right axis value"=w269, "Left axis value"=w270, "RobotDriveDevRef"=w259) -> ("Motor Values"=w258:dbl[])  [unwired: 3 in, 2 out]
      }
    }
    n113 = Unbundle By Name(w126) -> ("Drive Base Mode"=w127:T3)
    n114 = call-poly <vilib>:"NT Write Value.vi"("Numeric Array"=w118, "Name"="RobotDrive Motors") -> ()  [unwired: 9 in, 1 out]
  }
  n115 = Obtain Notifier(name (unnamed)="Shooter Control", notification data type=T2 {"Fire"=FALSE, "Open Claw"=FALSE}) -> (notifier out=w17:refnum<notifier>, error out=w16:errorcluster)  [unwired: 2 in, 1 out]
  n116 = call <vilib>:"WPI_SolenoidRefNum Registry Get.vi"("refnum name"=T1 "PCM - Shooter" ("Device Name")) -> ("error out"=w20:errorcluster, "SolenoidDevRef"=w21:T30)  [unwired: 9 in]
  n117 = call <vilib>:"WPI_SolenoidRefNum Registry Get.vi"("error in (no error)"=w20, "refnum name"=T1 "PCM - Intake Open/Close" ("Device Name")) -> ("error out"=w23:errorcluster, "SolenoidDevRef"=w24:T30)  [unwired: 8 in]
  n118 = while {
    tunnel: w24 -> [w315]
    tunnel: w23 -> [w314]
    tunnel: w21 -> [w313]
    tunnel: w17 -> [w311]
    tunnel: w16 -> [w310]
    stop <- FALSE ("stop") stop-if-true
    # "Set 'Fire Ready' Indicator"
    # "Conditions to allow the shooter to fire."
    # "Shooter Control"
    n119 = Wait on Notification(notifier=w311, timeout in ms (-1)=50, error in (no error)=w310) -> (notification=w307:T2, timed out?=w306:bool)  [unwired: 1 in, 2 out]
    n120 = call-poly <vilib>:"NT Read Value.vi"("Default Value"=75.0, "Name"="/Robot Parameters/Shooter Parameters/Pressure threshold for shooting (PSI)") -> ("Numeric"=w305:dbl)  [unwired: 8 in, 1 out]
    n121 = call-poly <vilib>:"NT Read Value.vi"("Default Value"=120.0, "Name"="/Robot Parameters/Shooter Parameters/Arm angle threshold for shooting (90°-180°)") -> ("Numeric"=w300:dbl)  [unwired: 8 in, 1 out]
    n122 = global read "Global Variables.vi" "Air Pressure"() -> (w312:dbl)
    n123 = global read "Global Variables.vi" "Arm Angle"() -> (w301:dbl)
    n124 = call-poly <vilib>:"NT Read Value.vi"("Default Value"=300.0, "Name"="/Robot Parameters/Shooter Parameters/Shoot Solenoid Time (ms)") -> ("Numeric"=w290:dbl)  [unwired: 8 in, 1 out]
    n125 = call-poly <vilib>:"NT Read Value.vi"("Default Value"=200.0, "Name"="/Robot Parameters/Shooter Parameters/Open Claw Time (ms)") -> ("Numeric"=w289:dbl)  [unwired: 8 in, 1 out]
    n126 = Greater Or Equal?(x=w312, y=w305) -> (x >= y?=w302:bool)
    n127 = Greater Or Equal?(x=w301, y=w300) -> (x >= y?=w299:bool)
    n128 = Compound Arithmetic op=AND(w302, w299) -> (w309:bool)
    n129 = global write "Global Variables.vi" "Fire Ready"(w309) -> ()
    n130 = To Unsigned Long Integer(number=w290) -> (unsigned 32bit integer=w303:u32)
    n131 = To Unsigned Long Integer(number=w289) -> (unsigned 32bit integer=w304:u32)
    n132 = case shown="False" w306 {
      tunnel: w315 -> [w325 _]
      tunnel: w314 -> [w324 _]
      tunnel: w313 -> [w323 _]
      tunnel: w309 -> [w321 _]
      tunnel: w307 -> [w319 _]
      tunnel: w304 -> [w318 _]
      tunnel: w303 -> [w317 _]
      frame False {
        n133 = Unbundle By Name(w319) -> ("Fire"=w320:bool)
        n134 = call "Rising Edge Detector.vi"("Input"=w320) -> ("Rising Edge Detected"=w322:bool)
        n135 = And(x=w322, y=w321) -> (x .and. y?=w326:bool)
        n136 = case shown="True" w326 {
          tunnel: w325 -> [w336 w349]
          tunnel: w324 -> [w333 w348]
          tunnel: w323 -> [w334 w347]
          tunnel: w319 -> [w331 _]
          tunnel: w318 -> [_ w339]
          tunnel: w317 -> [_ w338]
          frame False {
            n137 = Unbundle By Name(w331) -> ("Open Claw"=w327:bool)
            n138 = call-poly <vilib>:"WPI_SolenoidSet.vi"("error in (no error)"=w333, "Value"=WPI_SolenoidValue."Off", "SolenoidDevRef"=w334) -> ("error out"=w332:errorcluster)  [unwired: 7 in, 1 out]
            n139 = Select(t=WPI_SolenoidValue."On" ("Value"), s=w327, f=WPI_SolenoidValue."Off" ("Value")) -> (s? t:f=w330:T32)
            n140 = call-poly <vilib>:"WPI_SolenoidSet.vi"("error in (no error)"=w332, "Value"=w330, "SolenoidDevRef"=w336) -> ()  [unwired: 7 in, 2 out]
          }
          frame True {
            n141 = flat-sequence {
              tunnel: w349 -> [w355]
              tunnel: w348 -> [w354]
              tunnel: [w353] -> w345
              tunnel: [w352] -> w343
              tunnel: w339 -> [w350]
              tunnel: w347 -> [w362]
              tunnel: [w361] -> w346
              tunnel: w345 -> [w360]
              tunnel: [w360] -> w344
              tunnel: w343 -> [w359]
              tunnel: [w358] -> w342
              tunnel: w338 -> [w356]
              tunnel: [w356] -> w337
              tunnel: w346 -> [w368]
              tunnel: w344 -> [w364]
              tunnel: w342 -> [w367]
              tunnel: [w366] -> w341
              tunnel: [w364] -> w340
              tunnel: w337 -> [w363]
              tunnel: w341 -> [w371]
              tunnel: w340 -> [w369]
              frame #0 {
                # "Open Claw"
                n142 = call-poly <vilib>:"WPI_SolenoidSet.vi"("error in (no error)"=w354, "Value"=WPI_SolenoidValue."On", "SolenoidDevRef"=w355) -> ("error out"=w352:errorcluster, "SolenoidDevRef"=w353:T30)  [unwired: 7 in]
                n143 = Wait (ms)(milliseconds to wait=w350) -> ()  [unwired: 1 out]
              }
              frame #1 {
                # "Fire Shooter"
                n144 = call-poly <vilib>:"WPI_SolenoidSet.vi"("error in (no error)"=w359, "Value"=WPI_SolenoidValue."On", "SolenoidDevRef"=w362) -> ("error out"=w358:errorcluster, "SolenoidDevRef"=w361:T30)  [unwired: 7 in]
                n145 = Wait (ms)(milliseconds to wait=w356) -> ()  [unwired: 1 out]
              }
              frame #2 {
                # "Retract Shooter"
                n146 = call-poly <vilib>:"WPI_SolenoidSet.vi"("error in (no error)"=w367, "Value"=WPI_SolenoidValue."Off", "SolenoidDevRef"=w368) -> ("error out"=w366:errorcluster)  [unwired: 7 in, 1 out]
                n147 = Wait (ms)(milliseconds to wait=w363) -> ()  [unwired: 1 out]
              }
              frame #3 {
                # "Close Claw"
                n148 = call-poly <vilib>:"WPI_SolenoidSet.vi"("error in (no error)"=w371, "Value"=WPI_SolenoidValue."Off", "SolenoidDevRef"=w369) -> ()  [unwired: 7 in, 2 out]
              }
            }
          }
        }
      }
      frame True {
      }
    }
  }
  n149 = call <vilib>:"WPI_SwitchRefNum Registry Get.vi"("refnum name"=T1 "Lock Disengaged" ("Device Name")) -> ("error out"=w28:errorcluster, "SwitchDevRef"=w35:T33)  [unwired: 9 in]
  n150 = call <vilib>:"WPI_MotorControlRefNum Registry Get.vi"("refnum name"=T1 "Arm Motor - Closed Loop Control" ("Device Name")) -> ("error out"=w34:errorcluster, "MotorControlDevRef"=w33:T10)  [unwired: 9 in]
  n151 = call <vilib>:"WPI_AnalogChannelRefNum Registry Get.vi"("refnum name"=T1 "Analog Arm Position Sensor" ("Device Name")) -> ("error out"=w31:errorcluster, "AIDeviceRef"=w32:T24)  [unwired: 9 in]
  n152 = call <vilib>:"WPI_SolenoidRefNum Registry Get.vi"("refnum name"=T1 "PCM - Arm Lock" ("Device Name")) -> ("error out"=w26:errorcluster, "SolenoidDevRef"=w27:T30)  [unwired: 9 in]
  n153 = while {
    stop <- FALSE stop-if-true
    # "If we have a persistence file, populate the table with the variables"
    n154 = call <vilib>:"Dflt Data Dir.vi"() -> ("App:Default Data Directory"=w372:path)
    n155 = Build Path(base path=w372, name or relative path="persistent_perm.ini") -> (appended path=w376:path)
    n156 = call <vilib>:"Open Config Data.vi"("create file if necessary (T)"=FALSE, "configuration file path"=w376) -> ("error out"=w374:errorcluster, "refnum"=w378:T35)  [unwired: 7 in, 1 out]
    n157 = call-poly <vilib>:"Read Key.vi"("section"="NT Version", "error in (no error)"=w374, "key"="NT version" ("section"), "refnum"=w378) -> ("error out"=w373:errorcluster, "value"=w381:string, "refnum out"=w382:T35)  [unwired: 4 in, 1 out]
    n158 = case shown="\"3.0\", Default" w381 {
      tunnel: w382 -> [w387 w392]
      tunnel: "Types" ("section") -> [_ w390]
      tunnel: [w387 w389] -> w384
      tunnel: w373 -> [_ _]
      frame "" {
      }
      frame "3.0", Default {
        n159 = call <vilib>:"Get Key Names.vi"("section"=w390, "refnum"=w392) -> ("key names"=w388:string[], "refnum out"=w391:T35)  [unwired: 6 in, 2 out]
        n160 = for {
          tunnel: w388 -> [w395] mode=indexing
          shift-right: [w397] -> w389
          shift-left: w391 -> [w401]
          tunnel: w390 -> [w396]
          n161 = call-poly <vilib>:"Read Key.vi"("section"=w396, "key"=w395, "refnum"=w401) -> ("value"=w400:string, "refnum out"=w399:T35)  [unwired: 5 in, 2 out]
          n162 = case shown="\"Boolean Array\"" w400 {
            tunnel: w399 -> [w403 w408 w413 w418 w424 w430 w436 w442]
            tunnel: "Values" ("section") -> [_ w407 w410 w417 w422 w429 w434 w441]
            tunnel: [w403 w406 w412 w416 w423 w427 w435 w440] -> w397
            tunnel: w395 -> [_ w404 w409 w414 w421 w428 w433 w439]
            tunnel: [_ w404 w409 w414 w421 w428 w433 w439] -> w394
            tunnel: [errorcluster {"status"=TRUE, "code"=20, "source"=""} ("error in") _ _ _ _ _ _ _] -> w393
            frame Default {
            }
            frame "Boolean" {
              n163 = call-poly <vilib>:"Read Key.vi"("section"=w407, "key"=w404, "refnum"=w408) -> ("value"=w405:bool, "refnum out"=w406:T35)  [unwired: 5 in, 2 out]
              n164 = call-poly <vilib>:"NT Write Value.vi"("Boolean"=w405, "Name"=w404) -> ()  [unwired: 9 in, 1 out]
            }
            frame "Number" {
              n165 = call-poly <vilib>:"Read Key.vi"("section"=w410, "key"=w409, "refnum"=w413) -> ("value"=w411:dbl, "refnum out"=w412:T35)  [unwired: 5 in, 2 out]
              n166 = call-poly <vilib>:"NT Write Value.vi"("Numeric"=w411, "Name"=w409) -> ()  [unwired: 9 in, 1 out]
            }
            frame "String" {
              n167 = call-poly <vilib>:"Read Key.vi"("section"=w417, "key"=w414, "refnum"=w418) -> ("value"=w415:string, "refnum out"=w416:T35)  [unwired: 5 in, 2 out]
              n168 = call-poly <vilib>:"NT Write Value.vi"("String"=w415, "Name"=w414) -> ()  [unwired: 9 in, 1 out]
            }
            frame "Raw" {
              n169 = call-poly <vilib>:"Read Key.vi"("section"=w422, "key"=w421, "refnum"=w424) -> ("value"=w420:string, "refnum out"=w423:T35)  [unwired: 5 in, 2 out]
              n170 = call <vilib>:"base64_fast_decode.vi"("string in (base64-encoded)"=w420) -> ("string out (decoded)"=w419:string)  [unwired: 9 in, 1 out]
              n171 = call-poly <vilib>:"NT Write Value.vi"("Raw"=w419, "Name"=w421) -> ()  [unwired: 9 in, 1 out]
            }
            frame "Boolean Array" {
              # "Parse Bool[]"
              n172 = call-poly <vilib>:"Read Key.vi"("section"=w429, "key"=w428, "refnum"=w430) -> ("value"=w426:string, "refnum out"=w427:T35)  [unwired: 5 in, 2 out]
              n173 = call <vilib>:"Parse Persisted Bool Array.vi"("file string value"=w426) -> ("Array of Booleans"=w425:bool[])  [unwired: 9 in, 1 out]
              n174 = call-poly <vilib>:"NT Write Value.vi"("Boolean Array"=w425, "Name"=w428) -> ()  [unwired: 9 in, 1 out]
            }
            frame "Numeric Array" {
              n175 = call-poly <vilib>:"Read Key.vi"("section"=w434, "key"=w433, "refnum"=w436) -> ("value"=w432:string, "refnum out"=w435:T35)  [unwired: 5 in, 2 out]
              n176 = call <vilib>:"Parse Persisted Num Array.vi"("file string value"=w432) -> ("Array of Booleans"=w431:dbl[])  [unwired: 9 in, 1 out]
              n177 = call-poly <vilib>:"NT Write Value.vi"("Numeric Array"=w431, "Name"=w433) -> ()  [unwired: 9 in, 1 out]
            }
            frame "String Array" {
              n178 = call-poly <vilib>:"Read Key.vi"("section"=w441, "key"=w439, "refnum"=w442) -> ("value"=w438:string, "refnum out"=w440:T35)  [unwired: 5 in, 2 out]
              n179 = call <vilib>:"Decode String Array.vi"("Encoded String"=w438) -> ("Strings"=w437:string[])  [unwired: 10 in]
              n180 = call-poly <vilib>:"NT Write Value.vi"("String Array"=w437, "Name"=w439) -> ()  [unwired: 9 in, 1 out]
            }
          }
          n181 = call <vilib>:"NT Update Persistence.vi"("error in"=w393, "Name"=w394) -> ()  [unwired: 9 in, 1 out]
        }
      }
    }
    n182 = Wait (ms)(milliseconds to wait=u32 1000) -> ()  [unwired: 1 out]
    n183 = call <vilib>:"Close Config Data.vi"("refnum"=w384) -> ()  [unwired: 9 in, 2 out]
  }
  n184 = while {
    tunnel: w35 -> [w467]
    tunnel: w34 -> [w466]
    tunnel: w33 -> [w465]
    tunnel: w32 -> [w461]
    tunnel: w31 -> [w448]
    tunnel: w28 -> [w464]
    tunnel: w27 -> [w463]
    tunnel: w26 -> [w462]
    stop <- FALSE stop-if-true
    # "Make it 'False' if unlocked"
    # "Returns 'True' if unlocked"
    # "Set Arm Lock"
    # "Arm Control"
    n185 = call <vilib>:"WPI_SwitchGetLimitValue.vi"("error in (no error)"=w464, "SwitchDevRef"=w467) -> ("Switch Pressed"=w444:bool)  [unwired: 7 in, 2 out]
    n186 = Not(x=w444) -> (.not. x?=w450:bool)
    n187 = global read "Global Variables.vi" "Arm Control"() -> (w468:T37)
    n188 = call-poly <vilib>:"NT Write Value.vi"("Boolean"=w444, "Name"="Arm Unlocked?") -> ()  [unwired: 9 in, 1 out]
    n189 = Unbundle By Name(w468) -> ("Arm Mode"=w443:T36)
    n190 = call "Arm - In Position Detector.vi"("error in (no error)"=w448, "Current Arm Mode"=w443, "AIDeviceRef"=w461) -> ("Current Angle"=w445:dbl, "Set Angle"=w446:dbl, "Disable Motor"=w449:bool, "Set Lock"=w447:bool)  [unwired: 4 in, 1 out]
    n191 = Equal?(x=w443, y=Arm_Mode_TypeDef."Disabled") -> (x = y?=w454:bool)
    n192 = Select(t=WPI_SolenoidValue."Forward" ("Value"), s=w447, f=WPI_SolenoidValue."Reverse" ("Value")) -> (s? t:f=w453:T32)
    n193 = Compound Arithmetic op=OR(w454, w450, w449) -> (w456:bool)
    n194 = call-poly <vilib>:"WPI_SolenoidSet.vi"("error in (no error)"=w462, "Value"=w453, "SolenoidDevRef"=w463) -> ()  [unwired: 7 in, 2 out]
    n195 = call "Falling Edge Detector.vi"("Input"=w456) -> ("Falling Edge Detected"=w459:bool)
    n196 = case shown="False" w456 {
      tunnel: w466 -> [w484 w493]
      tunnel: w465 -> [w485 w491]
      tunnel: w446 -> [w489 _]
      tunnel: w445 -> [w488 _]
      tunnel: w459 -> [w486 _]
      frame False {
        # "Arm Motor Enabled"
        n197 = call "Get NT PID Parameter.vi"("NT Path"="/Robot Parameters/Arm Parameters/Arm Motor PID Gains") -> ("PID Gains"=w481:T28)
        n198 = call-poly <vilib>:"PID.vi"("reinitialize? (F)"=w486, "output range"=cluster{"output high":dbl, "output low":dbl} {"output high"=1.0, "output low"=-1.0}, "PID gains"=w481, "process variable"=w488, "setpoint"=w489) -> ("output"=w482:dbl)  [unwired: 5 in, 1 out]
        n199 = call <vilib>:"WPI_CANTalonSRX_ChangeMode.vi"("error in (no error)"=w484, "Output"=w482, "Control Mode"=WPI_CANTalonSRX_APIControlMode."Percent VBus", "CAN Talon SRX Ref"=w485) -> ()  [unwired: 6 in, 2 out]
      }
      frame True {
        # "Arm Motor Disabled"
        n200 = call <vilib>:"WPI_CANTalonSRX_ChangeMode.vi"("error in (no error)"=w493, "Output"=0.0, "Control Mode"=WPI_CANTalonSRX_APIControlMode."Percent VBus", "CAN Talon SRX Ref"=w491) -> ()  [unwired: 6 in, 2 out]
      }
    }
    n201 = case shown="\"Cross Defense\"" w443 {
      tunnel: ["Invalid" "Disabled" "Locked" "Shoot Batter" "Shoot Close" "Cross Defense" "Human Player Load" "Low Bar / Goal" "Manual"] -> w457
      frame "Unknown", Default {
      }
      frame "Disabled" {
      }
      frame "Locked" {
      }
      frame "Shoot Batter" {
      }
      frame "Shoot Close" {
      }
      frame "Cross Defense" {
      }
      frame "Human Player Load" {
      }
      frame "Low Bar / Goal" {
      }
      frame "Manual" {
      }
    }
    n202 = Wait (ms)(milliseconds to wait=u32 20) -> ()  [unwired: 1 out]
    n203 = global write "Global Variables.vi" "Current Arm Mode"(w443) -> ()
    n204 = call-poly <vilib>:"NT Write Value.vi"("String"=w457, "Name"="Arm - Mode") -> ()  [unwired: 9 in, 1 out]
  }
  n205 = while {
    stop <- FALSE stop-if-true
    # "Operator Interface Control Board"
    n206 = global read "Global Variables.vi" "Fire Ready"() -> (w508:bool)
    n207 = global read "Global Variables.vi" "Arm Mode LEDs"() -> (w505:T40)
    n208 = Unbundle By Name(w505) -> ("Shoot Batter"=w504:bool, "Shoot Close"=w503:bool, "Shoot Far"=w502:bool, "Human Player Load"=w501:bool, "Low Bar / Goal"=w500:bool, "Manual"=w499:bool)
    n209 = Bundle By Name(cluster=T39 {"LED 0"=FALSE, "LED 1"=FALSE, "LED 2"=FALSE, "LED 3"=FALSE, "LED 4"=FALSE, "LED 5"=FALSE, "LED 6"=FALSE, "LED 7"=FALSE, "LED 8"=FALSE, "LED 9"=FALSE, "LED 10"=FALSE, "LED 11"=FALSE, "LED 12"=FALSE, "LED 13"=FALSE, "LED 14"=FALSE, "LED 15"=FALSE} ("LED Outputs"), "LED 0"=w508, "LED 1"=w504, "LED 2"=w503, "LED 3"=w502, "LED 4"=w501, "LED 5"=w500, "LED 6"=w499) -> (w506:T39)
    n210 = call "OICB - Set PWM.vi"("PWM Outputs"=T38 {"PWM 0"=0, "PWM 1"=0, "PWM 2"=0, "PWM 3"=0, "PWM 4"=0, "PWM 5"=0, "PWM 6"=0, "PWM 7"=0, "PWM 8"=0, "PWM 9"=0, "PWM 10"=0}) -> ()  [unwired: 10 in, 1 out]
    n211 = call "OICB - Get Switches.vi"() -> ("Switch Inputs"=w509:T26)  [unwired: 10 in, 1 out]
    n212 = call "OICB - Get Analog.vi"() -> ("Analog"=w495:T41)  [unwired: 10 in, 1 out]
    n213 = call "OICB - Set LED's.vi"("LED Outputs"=w506) -> ()  [unwired: 10 in, 1 out]
    n214 = global write "Global Variables.vi" "Analog Inputs"(w495) -> ()
    n215 = Wait (ms)(milliseconds to wait=u32 20) -> ()  [unwired: 1 out]
    n216 = Unbundle By Name(w495) -> ("ANA 0"=w496:u8)
    n217 = call "Autonomous - Get Mode.vi"("Autonomous Selector Value"=w496) -> ("Autonomous Mode"=w494:T42)  [unwired: 1 in]
    n218 = global write "Global Variables.vi" "Autonomous Mode"(w494) -> ()
    n219 = global write "Global Variables.vi" "Switch Inputs"(w509) -> ()
    n220 = call-poly <vilib>:"NT Write Value.vi"("Numeric"=w494, "Name"="Autonomous Mode") -> ()  [unwired: 9 in, 1 out]
  }
